vi "IsTimeString.vi"(0 "Input String":string) -> (7 "Number String":string, 8 "Numeric Value":dbl, 10 "Is Time String":bool)   [LabVIEW 2013]
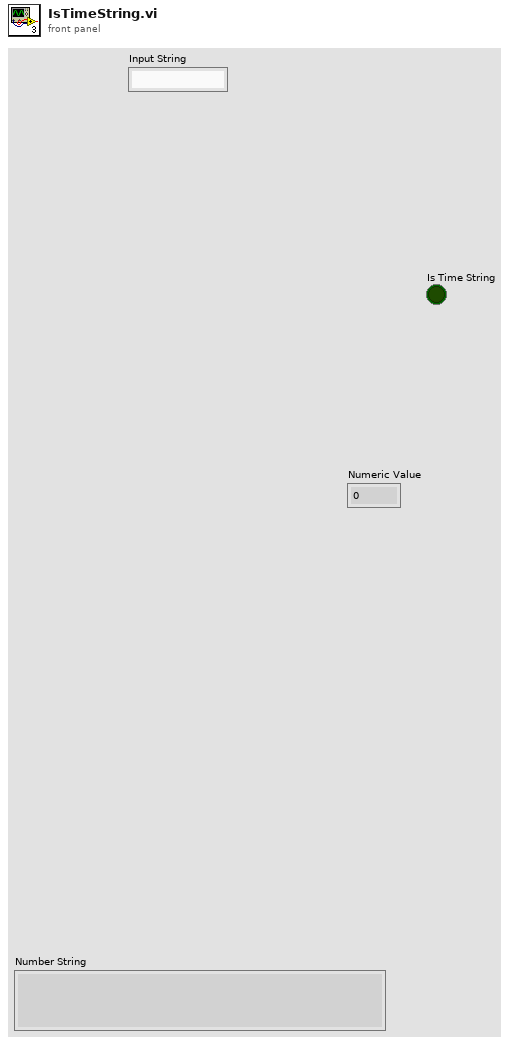
[diagram p1: front panel]
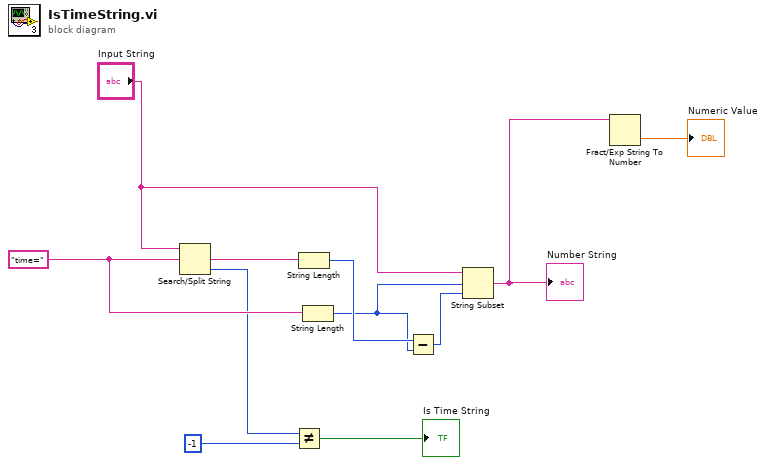
[diagram p0: block diagram]
diagram:
  w10 = "time=" ("search string/char (-)")
  n1 = Search/Split String(string="Input String", search string/char (-)=w10) -> (match + rest of string=w11:string, offset of match=w6:i32)  [unwired: 1 in, 1 out]
  n2 = Not Equal?(x=w6, y=-1) -> (x != y?=→"Is Time String":bool)
  n3 = String Length(string=w11) -> (length=w9:i32)
  n4 = String Length(string=w10) -> (length=w8:i32)
  n5 = Subtract(x=w9, y=w8) -> (x-y=w7:i32)
  n6 = String Subset(string="Input String", offset (0)=w8, length (rest)=w7) -> (substring=w1:string)
  "Number String" <- w1
  n7 = Fract/Exp String To Number(string=w1) -> (number=→"Numeric Value":dbl)  [unwired: 3 in, 1 out]
